vi "Compare Display Parameters.vi"(0 "display parameters in":T1[](array[typedef])=[{"virtual channel"=0.0, "payload data type"=enum."Frame Start", "frame skip count"=0, "line skip count"=0, "pixel skip count"=0.0}, {"virtual channel"=0.0, "payload data type"=enum."Frame Start", "frame skip count"=0, "line skip count"=0, "pixel skip count"=0.0}, {"virtual channel"=0.0, "payload data type"=enum."Frame Start", "frame skip count"=0, "line skip count"=0, "pixel skip count"=0.0}, {"virtual channel"=0.0, "payload data type"=enum."Frame Start", "frame skip count"=0, "line skip count"=0, "pixel skip count"=0.0}, {"virtual channel"=0.0, "payload data type"=enum."Frame Start", "frame skip count"=0, "line skip count"=0, "pixel skip count"=0.0}, {"virtual channel"=0.0, "payload data type"=enum."Frame Start", "frame skip count"=0, "line skip count"=0, "pixel skip count"=0.0}, {"virtual channel"=0.0, "payload data type"=enum."Frame Start", "frame skip count"=0, "line skip count"=0, "pixel skip count"=0.0}, {"virtual channel"=0.0, "payload data type"=enum."Frame Start", "frame skip count"=0, "line skip count"=0, "pixel skip count"=0.0}], 5 "channel selector":fxp<+,3,3>, 7 "current state":T3) -> (4 "equal":bool)   [LabVIEW 2020, in "GettingStarted_Common_148X_FPGA.lvlib"]
uses:
  GettingStarted_Common_148X_FPGA.lvlib
  Types/Display Channel MUX State Data.ctl
  Types/Display Channel MUX State.ctl
  <instrlib>/FlexRIO/CSI-2/v2/FPGA/Types/Display Parameters.ctl
  <instrlib>/FlexRIO/CSI-2/v2/Common/Types/LLP Data Type.ctl
  <instrlib>/FlexRIO/CSI-2/v2/Common/NI CSI-2 API Common v2.lvlib
  <instrlib>/FlexRIO/CSI-2/v2/FPGA/NI CSI-2 API FPGA v2.lvlib
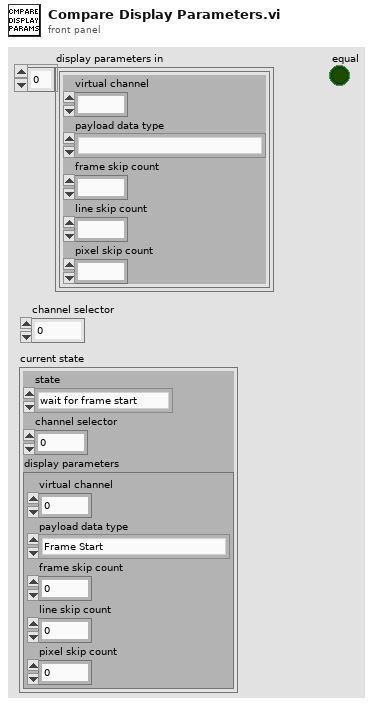
[diagram p1: front panel]
types:
  T1 = typedef "NI CSI-2 API FPGA v2.lvlib/Display Parameters.ctl" = cluster{"virtual channel":fxp<+,4,4>, "payload data type":T2, "frame skip count":u16, "line skip count":u8, "pixel skip count":fxp<+,5,5>}
  T2 = typedef "NI CSI-2 API Common v2.lvlib/LLP Data Type.ctl" = enum8{"Frame Start", "Frame End", "Line Start", "Line End", "End of Transmission", "Reserved 0", "Reserved 1", "Reserved 2", "Generic Short Packet 1", "Generic Short Packet 2", "Generic Short Packet 3", "Generic Short Packet 4", "Generic Short Packet 5", "Generic Short Packet 6", "Generic Short Packet 7", "Generic Short Packet 8", "Null", "Blanking Data", "Embedded 8-bit non Image Data", "Generic Long Packet 1", "Generic Long Packet 2", "Generic Long Packet 3", "Generic Long Packet 4", "Reserved 3", "YUV420 8-bit", "YUV420 10-bit", "Legacy YUV420 8-bit", "Reserved 4", "YUV420 8-bit Chroma Shifted", "YUV420 10-bit Chroma Shifted", "YUV422 8-bit", "YUV422 10-bit", "RGB444", "RGB555", "RGB565", "RGB666", "RGB888", "Reserved 5", "Reserved 6", "RAW 24", "RAW 6", "RAW 7", "RAW 8", "RAW 10", "RAW 12", "RAW 14", "RAW 16", "RAW 20", "User Defined 8-bit Data 1", "User Defined 8-bit Data 2", "User Defined 8-bit Data 3", "User Defined 8-bit Data 4", "User Defined 8-bit Data 5", "User Defined 8-bit Data 6", "User Defined 8-bit Data 7", "User Defined 8-bit Data 8", "USL Command", "Reserved 7", "Reserved 8", "Reserved 9", "Reserved 10", "Reserved 11", "Reserved 12", "LRTE EPD Spacer"}
  T3 = typedef "GettingStarted_Common_148X_FPGA.lvlib/Display Channel MUX State Data.ctl" = cluster{"state":T4, "channel selector":fxp<+,3,3>, "display parameters":T1}
  T4 = typedef "GettingStarted_Common_148X_FPGA.lvlib/Display Channel MUX State.ctl" = enum8{"wait for frame start", "wait for frame end", "clear pipeline and latch settings"}
  T5 = cluster{"virtual channel":bool, "payload data type":bool, "frame skip count":bool, "line skip count":bool, "pixel skip count":bool}
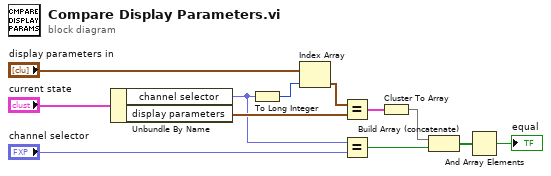
[diagram p0: block diagram]
diagram:
  n1 = Unbundle By Name("current state") -> ("channel selector"=w4:fxp<+,3,3>, "display parameters"=w5:T1)
  n2 = To Long Integer(number=w4) -> (32bit integer=w1:i32)
  n3 = Index Array(array="display parameters in", index=w1) -> (element=w6:T1)
  n4 = Equal?(x=w6, y=w5) -> (x = y?=w7:T5)
  n5 = Equal?(x=w4, y="channel selector") -> (x = y?=w8:bool)
  n6 = Cluster To Array(cluster=w7) -> (array=w9:bool[])
  n7 = Build Array (concatenate)(w9, w8) -> (w10:bool[])
  n8 = And Array Elements(Boolean array=w10) -> (logical AND=→"equal":bool)
